vi "GetCost.vi"(8 "error in (no error)":errorcluster, 11 "reference in":refnum<class "Rig.lvclass">) -> (0 "error out":errorcluster, 2 "Cost":dbl, 3 "reference in":refnum<class "Rig.lvclass">)   [LabVIEW 2020, in "Rig.lvclass"]
uses:
  Rig.lvclass
  Equipment_class/Equipment.lvclass
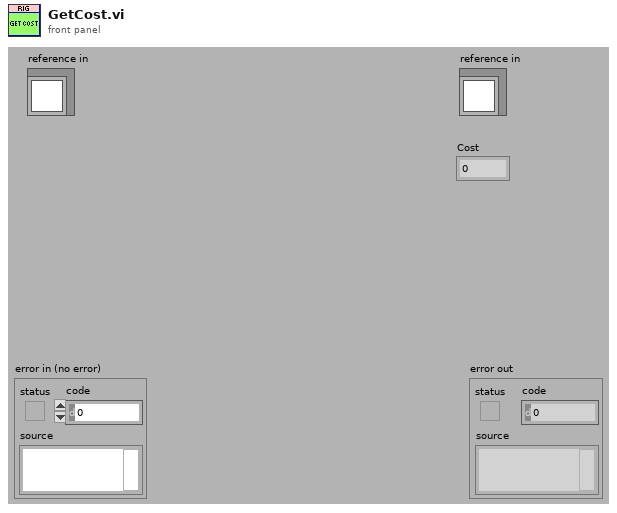
[diagram p1: front panel]
types:
  T1 = typedef "Rig.lvclass/ObjectAttributes.ctl" = cluster{"Children":refnum<class "Equipment.lvclass">[]}
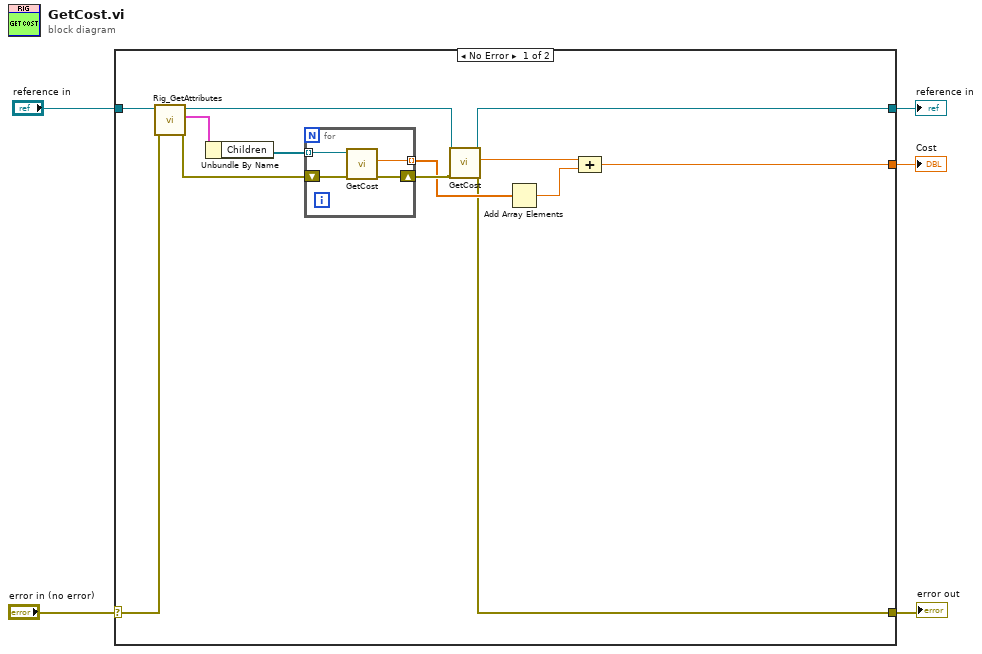
[diagram p0: block diagram]
diagram:
  n1 = case shown="No Error" "error in (no error)" {
    selector: "error in (no error)" -> [w18 w24]
    tunnel: [w10 w24] -> w4
    tunnel: [w6 w23] -> w2
    tunnel: "reference in" -> [w16 w23]
    tunnel: [w9 _] -> w1
    frame No Error {
      n2 = call "Rig_GetAttributes.vi"("error in (no error)"=w18, "reference in"=w16) -> ("error out"=w11:errorcluster, "Data"=w17:T1, "reference out"=w7:refnum<class "Rig.lvclass">)  [unwired: 6 in, 1 out]
      n3 = Unbundle By Name(w17) -> ("Children"=w15:refnum<class "Equipment.lvclass">[])
      n4 = for {
        tunnel: w15 -> [w22] mode=indexing
        shift-right: [w20] -> w14
        shift-left: w11 -> [w21]
        tunnel: [w19] -> w12 mode=indexing
        n5 = call-dynamic "GetCost.vi"("error in (no error)"=w21, "reference in"=w22) -> ("error out"=w20:errorcluster, "Cost"=w19:dbl)  [unwired: 7 in, 1 out]
      }
      n6 = call-parent "GetCost.vi"("error in (no error)"=w14, "reference in"=w7) -> ("error out"=w10:errorcluster, "Cost"=w13:dbl, "reference out"=w6:refnum<class "Rig.lvclass">)  [unwired: 7 in]
      n7 = Add Array Elements(numeric array=w12) -> (sum=w8:dbl)
      n8 = Compound Arithmetic op=ADD(w13, w8) -> (w9:dbl)
    }
    frame Error {
    }
  }
  "error out" <- w4
  "reference in" <- w2
  "Cost" <- w1
